vi "Add ACKs.vi"(8 "error in (no error)":errorcluster, 10 "Pending ACK":T1 {"Packet Identifier" format="%016b"}, 11 "Session in":refnum<class "Session.lvclass">) -> (0 "error out":errorcluster, 3 "Session out":refnum<class "Session.lvclass">)   [LabVIEW 2013, in "MQTT Base.lvlib" / "Session.lvclass"]
uses:
  Session.lvclass
  Pending ACKs -- cluster.ctl
  <vilib>/LabVIEW Open Source Project/MQTT Control Packets/Control Packets/ControlPacket/ControlPacket.lvclass
  Session.lvclass/Session.ctl
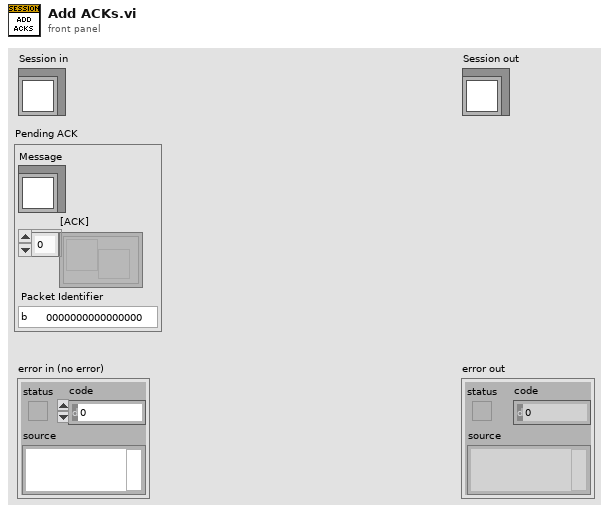
[diagram p1: front panel]
types:
  T1 = typedef "MQTT Base.lvlib/Session.lvclass/Pending ACKs -- cluster.ctl" = cluster{"Message":refnum<class "ControlPacket.lvclass">, "[ACK]":refnum<notifier>[], "Packet Identifier":u16}
  T2 = typedef "MQTT Base.lvlib/Session.lvclass/Session State -- cluster.ctl" = cluster{"CleanSession":bool, "Client ID":string, "Subscriptions":T3[], "Pending Transmissions":T5[], "Pending ACKs":T1[]}
  T3 = typedef "MQTT_Control_Packets.lvlib/SUBSCRIBE.lvclass/Topic Subscription -- cluster.ctl" = cluster{"Topic Filter":string, "QoS":T4}
  T4 = typedef "MQTT_Control_Packets.lvlib/ControlPacket.lvclass/QualityOfService -- enum.ctl" = enum16{"0 (At Most Once)", "1 (At Least Once)", "2 (Exactly Once)"}
  T5 = typedef "MQTT_Control_Packets.lvlib/ControlPacket.lvclass/Pending Transmission -- cluster.ctl" = cluster{"Message":refnum<class "ControlPacket.lvclass">, "QoS":T4, "Tx-Rx":bool}
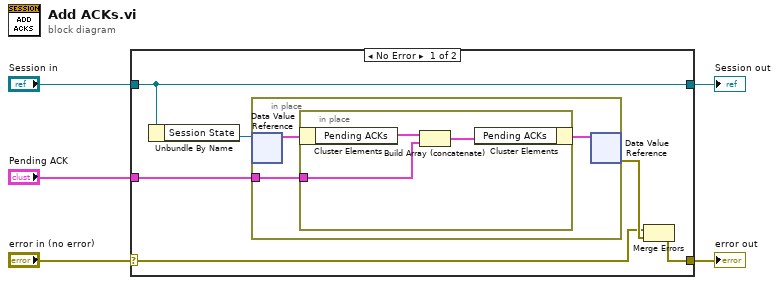
[diagram p0: block diagram]
diagram:
  n1 = case shown="No Error" "error in (no error)" {
    selector: "error in (no error)" -> [w7 w18]
    tunnel: [w6 w18] -> w4
    tunnel: [w11 w19] -> w2
    tunnel: "Session in" -> [w11 w19]
    tunnel: "Pending ACK" -> [w9 _]
    frame No Error {
      n2 = Unbundle By Name(w11) -> ("Session State"=w10:refnum<data-value>)
      n3 = in-place {
        in-place-border: w9 -> [w12]
        n4 = in-place-dvr #1(w10) -> (w14:T2)  [unwired: 1 out]
        n5 = in-place {
          in-place-border: w12 -> [w16]
          n6 = in-place-cluster #2(w14) -> ("Pending ACKs"=w17:T1[])
          n7 = Build Array (concatenate)(w17, w16) -> (w15:T1[])
          n8 = in-place-cluster #2("Pending ACKs"=w15) -> (w13:T2)
        }
        n9 = in-place-dvr #1(w13) -> (w8:errorcluster)  [unwired: 1 out]
      }
      n10 = Merge Errors(w7, w8) -> (w6:errorcluster)
    }
    frame Error {
    }
  }
  "error out" <- w4
  "Session out" <- w2
